vi "Resize 2D Array.vi"(9 "y dimension":i32=3, 10 "x dimension":i32=3, 11 "input array":dbl[][](array[numeric])=[[1.0, 2.0, 3.0, 4.0], [5.0, 6.0, 7.0, 8.0], [9.0, 10.0, 11.0, 12.0], [13.0, 14.0, 15.0, 16.0]]) -> (3 "output array":dbl[][](array[numeric]))   [LabVIEW 2024]
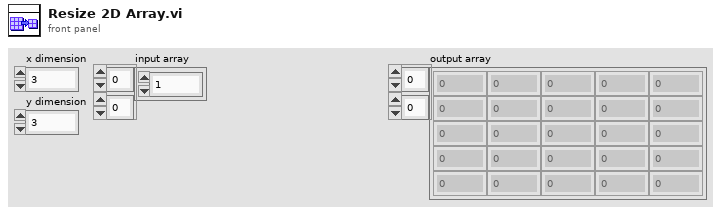
[diagram p1: front panel]
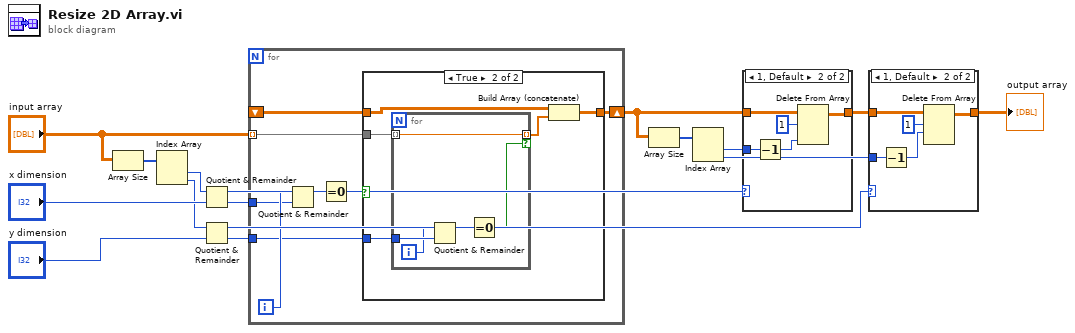
[diagram p0: block diagram]
diagram:
  n1 = Array Size(array="input array") -> (size(s)=w15:i32[])
  n2 = Index Array(array=w15) -> (element #1=w14:i32, element #2=w12:i32)  [unwired: 2 in]
  n3 = Quotient & Remainder(x=w14, y="x dimension") -> (x-y*floor(x/y)=w8:i32, floor(x/y)=w10:i32)
  n4 = Quotient & Remainder(x=w12, y="y dimension") -> (x-y*floor(x/y)=w3:i32, floor(x/y)=w9:i32)
  n5 = for {
    tunnel: "input array" -> [w21] mode=indexing
    tunnel: w10 -> [w23]
    tunnel: w9 -> [w19]
    shift-right: [w18] -> w2
    shift-left: _ -> [w17]
    i -> [w24]
    # "For each row"
    n6 = Quotient & Remainder(x=w24, y=w23) -> (x-y*floor(x/y)=w22:i32)  [unwired: 1 out]
    n7 = Equal To 0?(x=w22) -> (x = 0?=w20:bool)
    n8 = case shown="True" w20 {
      tunnel: w21 -> [_ w30]
      tunnel: w19 -> [_ w29]
      tunnel: [w25 w27] -> w18
      tunnel: w17 -> [w25 w26]
      frame False {
      }
      frame True {
        n9 = for {
          tunnel: w30 -> [w32] mode=indexing
          tunnel: w29 -> [w35]
          tunnel: [w32] -> w28 mode=indexing if=w31
          i -> [w34]
          n10 = Quotient & Remainder(x=w34, y=w35) -> (x-y*floor(x/y)=w33:i32)  [unwired: 1 out]
          n11 = Equal To 0?(x=w33) -> (x = 0?=w31:bool)
        }
        n12 = Build Array (concatenate)(w26, w28) -> (w27:dbl[][])
      }
    }
  }
  n13 = Array Size(array=w2) -> (size(s)=w7:i32[])
  n14 = Index Array(array=w7) -> (element #1=w6:i32, element #2=w4:i32)  [unwired: 2 in]
  n15 = case shown="1, Default" w8 {
    tunnel: w2 -> [w36 w41]
    tunnel: [w36 w40] -> w5
    tunnel: w6 -> [_ w37]
    frame 0 {
    }
    frame 1, Default {
      n16 = Decrement(x=w37) -> (x-1=w38:i32)
      n17 = Delete From Array(array=w41, length=1, index (col)=w38) -> (array with subset deleted=w40:dbl[][])  [unwired: 1 in, 1 out]
    }
  }
  n18 = case shown="1, Default" w3 {
    tunnel: w5 -> [w42 w47]
    tunnel: [w42 w46] -> w1
    tunnel: w4 -> [_ w44]
    frame 0 {
    }
    frame 1, Default {
      n19 = Decrement(x=w44) -> (x-1=w43:i32)
      n20 = Delete From Array(array=w47, length=1, index (row)=w43) -> (array with subset deleted=w46:dbl[][])  [unwired: 1 in, 1 out]
    }
  }
  "output array" <- w1
